vi "Status upload.vi"(8 "error in (no error)":errorcluster, 11 "Motor in":refnum<class "Motor.lvclass">) -> (0 "error out":errorcluster, 1 "error":bool, 2 "instructions":string[](array[string]), 3 "Motor out":refnum<class "Motor.lvclass">)   [LabVIEW 2018, in "Motor.lvclass"]
uses:
  Motor.lvclass
  Motor.lvclass/Motor.ctl
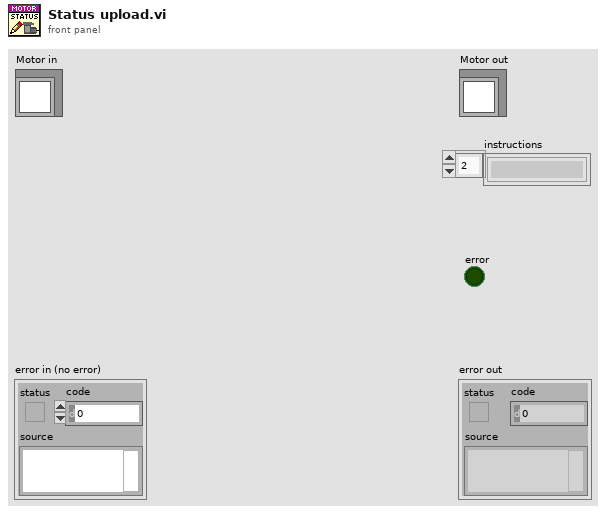
[diagram p1: front panel]
types:
  T1 = cluster{"mode":string, "condition":string, "position":string, "pos_name":string, "pos_id":string}
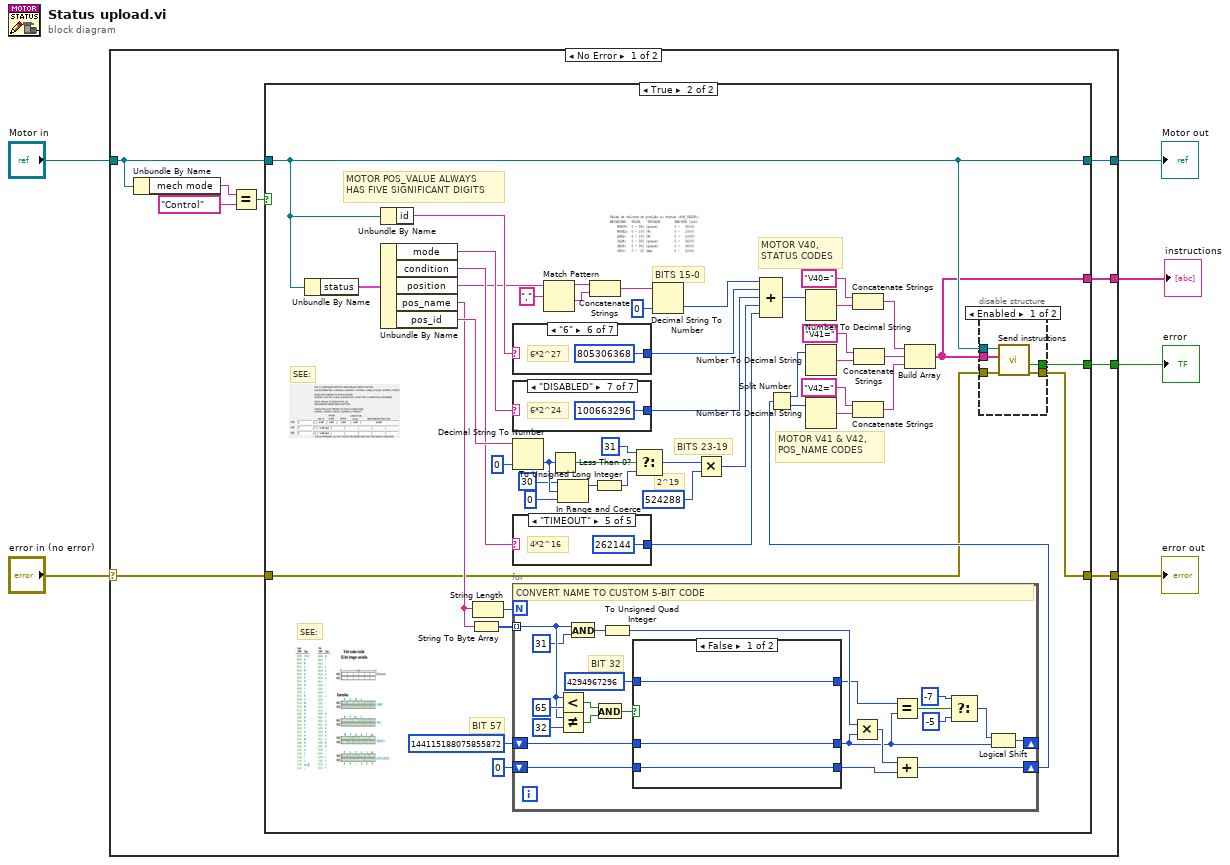
[diagram p0: block diagram]
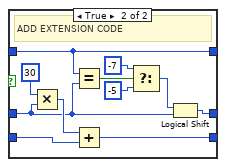
[diagram p4: hidden frame]
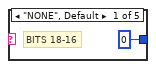
[diagram p5: hidden frame]
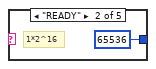
[diagram p6: hidden frame]
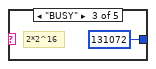
[diagram p7: hidden frame]
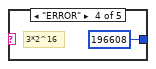
[diagram p8: hidden frame]
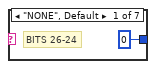
[diagram p9: hidden frame]
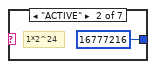
[diagram p10: hidden frame]
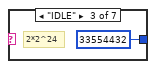
[diagram p11: hidden frame]
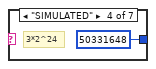
[diagram p12: hidden frame]
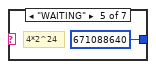
[diagram p13: hidden frame]
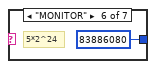
[diagram p14: hidden frame]
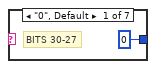
[diagram p15: hidden frame]
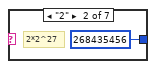
[diagram p16: hidden frame]
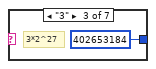
[diagram p17: hidden frame]
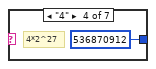
[diagram p18: hidden frame]
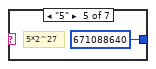
[diagram p19: hidden frame]
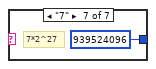
[diagram p20: hidden frame]
diagram:
  n1 = case shown="No Error" "error in (no error)" {
    selector: "error in (no error)" -> [w9 w128]
    tunnel: [w12 w128] -> w5
    tunnel: [w10 w129] -> w3
    tunnel: "Motor in" -> [w11 w129]
    tunnel: [w8 _] -> w2
    tunnel: [w7 _] -> w1
    frame No Error {
      n2 = Unbundle By Name(w11) -> ("mech mode"=w15:string)
      n3 = Equal?(x=w15, y="Control" ("GF mode")) -> (x = y?=w13:bool)
      n4 = case shown="True" w13 {
        tunnel: w11 -> [w17 w38]
        tunnel: [w16 w36] -> w12
        tunnel: [w17 w38] -> w10
        tunnel: w9 -> [w16 w37]
        tunnel: [_ w35] -> w8
        tunnel: [_ w34] -> w7
        frame False {
        }
        frame True {
          # "SEE:"
          # "SEE:"
          # "MOTOR V41 & V42, \nPOS_NAME CODES"
          # "BIT 57"
          # "MOTOR V40, \nSTATUS CODES"
          # "BITS 15-0"
          # "BITS 23-19"
          # "2^19"
          # "MOTOR POS_VALUE ALWAYS\nHAS FIVE SIGNIFICANT DIGITS"
          n5 = Unbundle By Name(w38) -> ("status"=w66:T1)
          n6 = Unbundle By Name(w38) -> ("id"=w63:string)
          n7 = Unbundle By Name(w66) -> ("mode"=w62:string, "condition"=w60:string, "position"=w24:string, "pos_name"=w55:string, "pos_id"=w61:string)
          n8 = String To Byte Array(string=w55) -> (unsigned byte array=w54:u8[])
          n9 = String Length(string=w55) -> (length=w56:i32)
          n10 = case shown="\"6\"" w63 {
            tunnel: [u32 0 ("y") u32 268435456 ("y") u32 402653184 ("y") u32 536870912 ("y") u32 671088640 ("y") u32 805306368 ("y") u32 939524096 ("y")] -> w59
            frame "0", Default {
              # "BITS 30-27"
            }
            frame "2" {
              # "2*2^27"
            }
            frame "3" {
              # "3*2^27"
            }
            frame "4" {
              # "4*2^27"
            }
            frame "5" {
              # "5*2^27"
            }
            frame "6" {
              # "6*2^27"
            }
            frame "7" {
              # "7*2^27"
            }
          }
          n11 = case shown="\"DISABLED\"" w62 {
            tunnel: [u32 0 ("y") u32 16777216 ("y") u32 33554432 ("y") u32 50331648 ("y") u32 671088640 ("y") u32 83886080 ("y") u32 100663296 ("y")] -> w58
            frame "NONE", Default {
              # "BITS 26-24"
            }
            frame "ACTIVE" {
              # "1*2^24"
            }
            frame "IDLE" {
              # "2*2^24"
            }
            frame "SIMULATED" {
              # "3*2^24"
            }
            frame "WAITING" {
              # "4*2^24"
            }
            frame "MONITOR" {
              # "5*2^24"
            }
            frame "DISABLED" {
              # "6*2^24"
            }
          }
          n12 = Decimal String To Number(string=w61, default (0L)=0 ("default (0 I32)")) -> (number=w28:i32)  [unwired: 1 in, 1 out]
          n13 = case shown="\"TIMEOUT\"" w60 {
            tunnel: [u32 0 ("y") u32 65536 ("y") u32 131072 ("y") u32 196608 ("y") u32 262144 ("y")] -> w57
            frame "NONE", Default {
              # "BITS 18-16"
            }
            frame "READY" {
              # "1*2^16"
            }
            frame "BUSY" {
              # "2*2^16"
            }
            frame "ERROR" {
              # "3*2^16"
            }
            frame "TIMEOUT" {
              # "4*2^16"
            }
          }
          n14 = for {
            N: w56 -> [_]
            tunnel: w54 -> [w87] mode=indexing
            shift-right: [w81] -> _
            shift-left: u64 144115188075855872 -> [w93]
            shift-right: [w80] -> w51
            shift-left: u64 0 -> [w88]
            # "BIT 32"
            # "CONVERT NAME TO CUSTOM 5-BIT CODE"
            n15 = Less?(x=w87, y=u8 65) -> (x < y?=w89:bool)
            n16 = Not Equal?(x=w87, y=u8 32) -> (x != y?=w91:bool)
            n17 = And(x=w87, y=u8 31) -> (x .and. y?=w85:u8)
            n18 = And(x=w89, y=w91) -> (x .and. y?=w90:bool)
            n19 = To Unsigned Quad Integer(1:w85) -> (0:w84:u64)
            n20 = case shown="False" w90 {
              tunnel: w93 -> [w96 w100]
              tunnel: w88 -> [w97 w106]
              tunnel: [w97 w105] -> w82
              tunnel: [w96 w104] -> w79
              tunnel: u64 4294967296 -> [w95 w98]
              tunnel: [w95 w98] -> w73
              frame False {
              }
              frame True {
                # "ADD EXTENSION CODE"
                n21 = Multiply(x=u64 30, y=w100) -> (x*y=w107:u64)
                n22 = Equal?(x=w98, y=w100) -> (x = y?=w101:bool)
                n23 = Add(x=w107, y=w106) -> (x+y=w105:u64)
                n24 = Select(t=i16 -7 ("y"), s=w101, f=i16 -5 ("y")) -> (s? t:f=w99:i16)
                n25 = Logical Shift(y=w99, x=w100) -> (x << y=w104:u64)
              }
            }
            n26 = Multiply(x=w84, y=w79) -> (x*y=w83:u64)
            n27 = Equal?(x=w73, y=w79) -> (x = y?=w78:bool)
            n28 = Add(x=w83, y=w82) -> (x+y=w80:u64)
            n29 = Select(t=i16 -7 ("y"), s=w78, f=i16 -5 ("y")) -> (s? t:f=w75:i16)
            n30 = Logical Shift(y=w75, x=w79) -> (x << y=w81:u64)
          }
          n31 = Match Pattern(string=w24, regular expression=",") -> (before substring=w22:string, after substring=w21:string)  [unwired: 1 in, 2 out]
          n32 = Less Than 0?(x=w28) -> (x < 0?=w32:bool)
          n33 = In Range and Coerce(upper limit=30 ("default (0 I32)"), x=w28, lower limit=0 ("default (0 I32)")) -> (coerced(x)=w25:i32)  [unwired: 1 out]
          n34 = Concatenate Strings(w22, w21) -> (w19:string)
          n35 = To Unsigned Long Integer(number=w25) -> (unsigned 32bit integer=w31:u32)
          n36 = Select(t=u32 31 ("default (0 I32)"), s=w32, f=w31) -> (s? t:f=w30:u32)
          n37 = Decimal String To Number(string=w19, default (0L)=u32 0 ("default (0 I32)")) -> (number=w18:u32)  [unwired: 1 in, 1 out]
          n38 = Multiply(x=w30, y=u32 524288) -> (x*y=w29:u32)
          n39 = Compound Arithmetic op=ADD(w18, w59, w58, w29, w57) -> (w48:u32)
          n40 = Split Number(x=w51) -> (hi(x)=w50:u32, lo(x)=w49:u32)
          n41 = Number To Decimal String(number=w48) -> (decimal integer string=w47:string)  [unwired: 1 in]
          n42 = Number To Decimal String(number=w50) -> (decimal integer string=w44:string)  [unwired: 1 in]
          n43 = Number To Decimal String(number=w49) -> (decimal integer string=w42:string)  [unwired: 1 in]
          n44 = Concatenate Strings("V40=", w47) -> (w40:string)
          n45 = Concatenate Strings("V42=", w42) -> (w39:string)
          n46 = Concatenate Strings("V41=", w44) -> (w41:string)
          n47 = Build Array(w40, w41, w39) -> (w34:string[])
          n48 = disable-structure shown="Enabled" {
            disable-tunnel: w38 -> [w71 _]
            disable-tunnel: w37 -> [w70 w72]
            disable-tunnel: [w69 w72] -> w36
            disable-tunnel: [w68 _] -> w35
            disable-tunnel: w34 -> [w67 _]
            frame Enabled {
              n49 = call-dynamic "Send instructions.vi"("error in (no error)"=w70, "instructions"=w67, "Motor in"=w71) -> ("error out"=w69:errorcluster, "error"=w68:bool)  [unwired: 4 in, 3 out]
            }
            frame Disabled {
            }
          }
        }
      }
    }
    frame Error {
    }
  }
  "error out" <- w5
  "Motor out" <- w3
  "error" <- w2
  "instructions" <- w1
